vi "Limit3DPointOutsideCuboid.vi"(10 "3D Cuboid":T2, 11 "3D Point":T1) -> (3 "Output Point":T1)   [LabVIEW 2023]
uses:
  3Dpoint.ctl
  3DCuboid.ctl
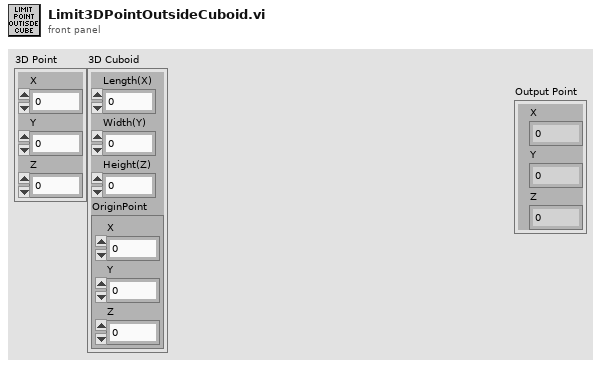
[diagram p1: front panel]
types:
  T1 = typedef "3Dpoint.ctl" = cluster{"X":dbl, "Y":dbl, "Z":dbl}
  T2 = typedef "3DCuboid.ctl" = cluster{"Length(X)":dbl, "Width(Y)":dbl, "Height(Z)":dbl, "OriginPoint":T1}
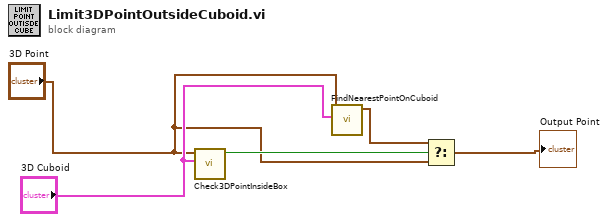
[diagram p0: block diagram]
diagram:
  n1 = call "Check3DPointInsideBox.vi"("3D Cuboid"="3D Cuboid", "3D Point"="3D Point") -> ("PointIsInsideCuboid"=w4:bool)  [unwired: 9 in]
  n2 = call "FindNearestPointOnCuboid.vi"("3D Cuboid"="3D Cuboid", "3D Point"="3D Point") -> ("Nearest Point"=w3:T1)  [unwired: 9 in]
  n3 = Select(t=w3, s=w4, f="3D Point") -> (s? t:f=→"Output Point":T1)
